vi "LockinDAQ.Generate.Waveforms.vi"(6 "Reset?":bool, 8 "error in (no error)":errorcluster, 11 "LockinDAQ":refnum<class "LockinDAQ.lvclass">) -> (0 "error out":errorcluster, 1 "REF []":waveform(dbl)[](array[waveform]), 2 "AO []":waveform(dbl)[](array[waveform]), 3 "LockinDAQ out":refnum<class "LockinDAQ.lvclass">)   [LabVIEW 2016, in "LockinDAQ.lvclass"]
uses:
  LockinDAQ.lvclass
  LockinDAQ.lvclass/LockinDAQ.ctl
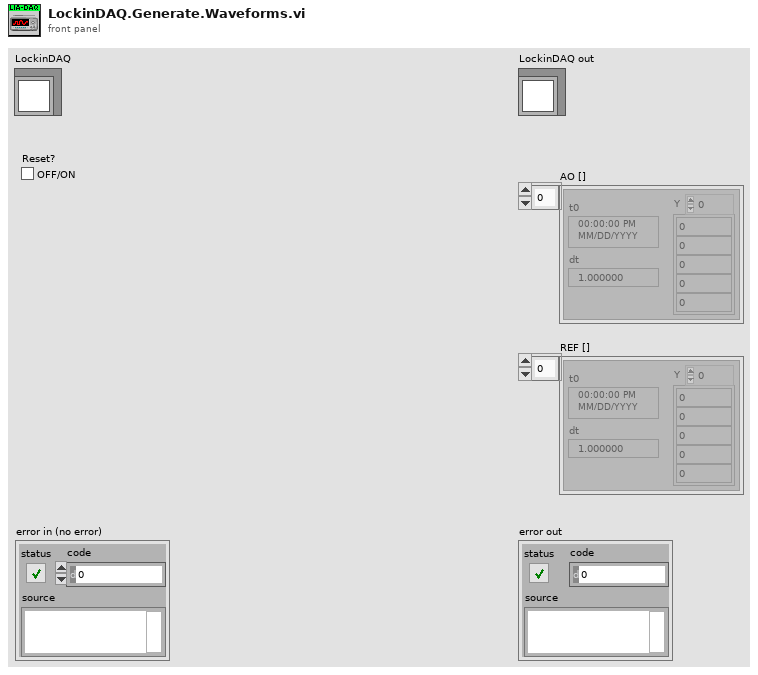
[diagram p1: front panel]
types:
  T1 = typedef "LockinDAQ.lvclass/AO-cluster.ctl" = cluster{"AO Amp (V)":T2, "AO DC (V)":T3, "AO f (Hz)":T4, "AO Phase (°)":T5, "Function":T6, "I+":bool[], "Sweeping":bool[]}
  T2 = typedef "LockinDAQ.lvclass/AO_Amp-array.ctl" = dbl[]
  T3 = typedef "LockinDAQ.lvclass/AO_DC-array.ctl" = dbl[]
  T4 = typedef "LockinDAQ.lvclass/AO_f-array.ctl" = dbl[]
  T5 = typedef "LockinDAQ.lvclass/AO_phi-array.ctl" = dbl[]
  T6 = typedef "LockinDAQ.lvclass/Function-array.ctl" = T7[]
  T7 = typedef "LockinDAQ.lvclass/Function-enum.ctl" = enum16{"Sine", "Triangle", "Square", "Sawtooth"}
  T8 = typedef "LockinDAQ.lvclass/REF-cluster.ctl" = cluster{"REF f (Hz)":T9, "REF phi (°)":T10}
  T9 = typedef "LockinDAQ.lvclass/REF_f-array.ctl" = dbl[]
  T10 = typedef "LockinDAQ.lvclass/REF_phi-array.ctl" = dbl[]
  T11 = typedef "LockinDAQ.lvclass/Sampling.ctl" = cluster{"Fs":dbl, "#s":i32}
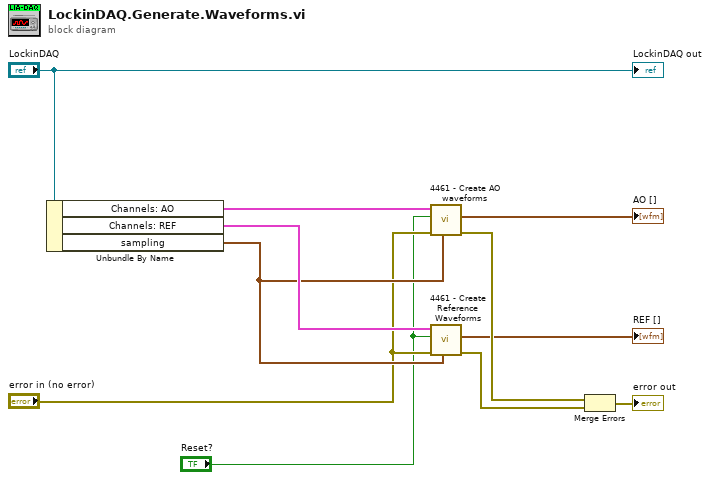
[diagram p0: block diagram]
diagram:
  n1 = Unbundle By Name("LockinDAQ") -> ("Channels: AO"=w5:T1, "Channels: REF"=w4:T8, "sampling"=w3:T11)
  n2 = call "4461 - Create AO waveforms.vi"("sampling"=w3, "error in (no error)"="error in (no error)", "reset signal"="Reset?", "AO"=w5) -> ("error out"=w11:errorcluster, "AO Array"=→"AO []":waveform(dbl)[])  [unwired: 4 in, 2 out]
  n3 = call "4461 - Create Reference Waveforms.vi"("sampling"=w3, "error in (no error)"="error in (no error)", "reset signal"="Reset?", "Lockin"=w4) -> ("error out"=w6:errorcluster, "AO Array"=→"REF []":waveform(dbl)[])  [unwired: 4 in, 2 out]
  n4 = Merge Errors(w11, w6) -> (→"error out":errorcluster)
  "LockinDAQ out" <- "LockinDAQ"
